vi "Read_Document.vi"(8 "error in (no error)":errorcluster caption="entrée d'erreur (pas d'erreur)", 11 "Firebase (Default) en entrée":refnum<class "Firebase Driver.lvclass">) -> (0 "error out":errorcluster caption="sortie d'erreur", 2 "Input.Name_Collection":string, 3 "Firebase (Default) en sortie":refnum<class "Firebase Driver.lvclass">)   [LabVIEW 2020, in "Library Instrument & Equipement.lvlib" / "Library FireBase.lvlib" / "Firebase Driver.lvclass"]
uses:
  Firebase Driver.lvclass
  Firebase Driver.lvclass/Firebase Driver.ctl
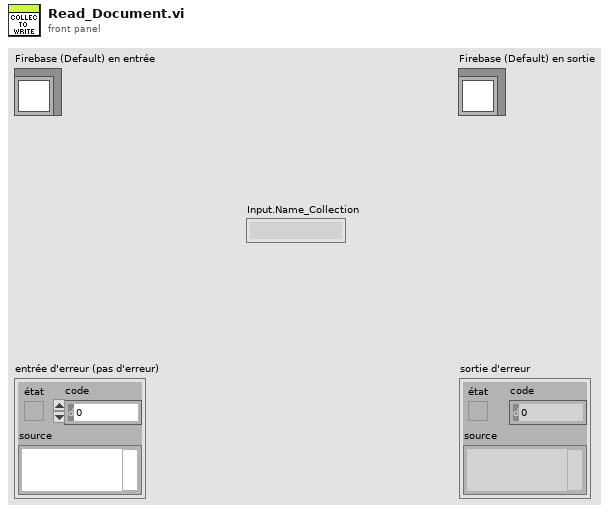
[diagram p1: front panel]
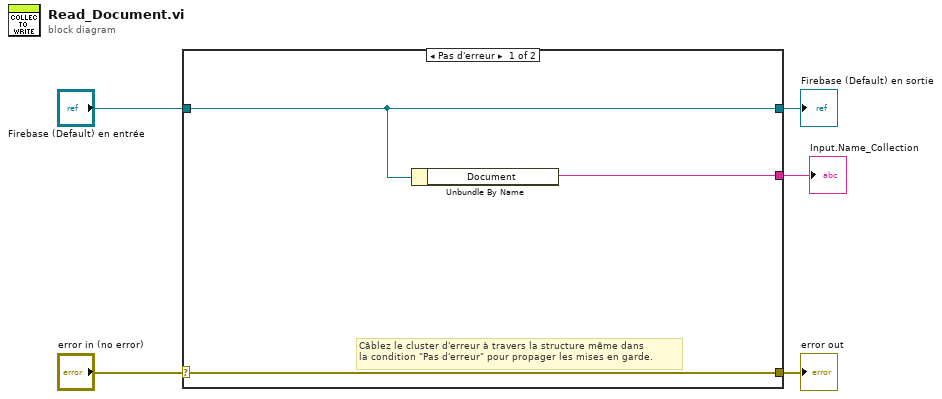
[diagram p0: block diagram]
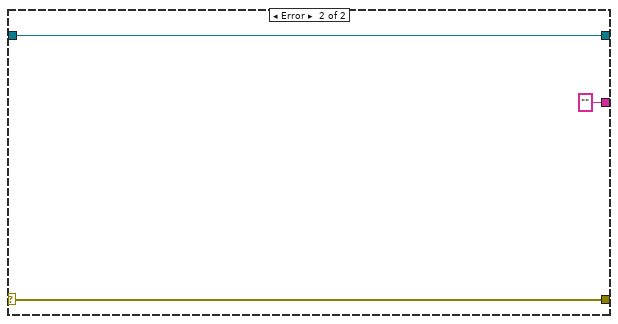
[diagram p2: hidden frame]
diagram:
  n1 = case shown="Pas d'erreur" "error in (no error)" {
    selector: "error in (no error)" -> [w8 w11]
    tunnel: [w8 w11] -> w4
    tunnel: [w7 w10] -> w2
    tunnel: "Firebase (Default) en entrée" -> [w7 w10]
    tunnel: [w6 "" ("Name_BDD")] -> w1
    frame No Error {
      # "Câblez le cluster d'erreur à travers la structure même dans\nla condition \"Pas d'erreur\" pour propager les mises en garde."
      n2 = Unbundle By Name(w7) -> ("Document"=w6:string)
    }
    frame Error {
    }
  }
  "error out" <- w4
  "Firebase (Default) en sortie" <- w2
  "Input.Name_Collection" <- w1
